vi "Keithley 6514 Zero Check Config.vi"(0 "Resource In":refnum<visa-resource-name>, 1 "Check For SCPI Errors? (T)":bool=TRUE, 7 "Zero Check (On:T)":bool=TRUE, 11 "error in (no error)":T1) -> (4 "Resource Out (dupl)":refnum<visa-resource-name>, 15 "error out":T1)   [LabVIEW 2009, in "Keithley 6514 LV 2009.lvlib"]
doc: "This VI for the Keithley 6514 Electrometer allows the operator to turn the 'Zero Check' function on or off.\n\n1 or True: Zero Check On\n0 or False: Zero Check Off"
uses:
  Keithley 6514 LV 2009.lvlib
panel:
  # "ON\nOFF"
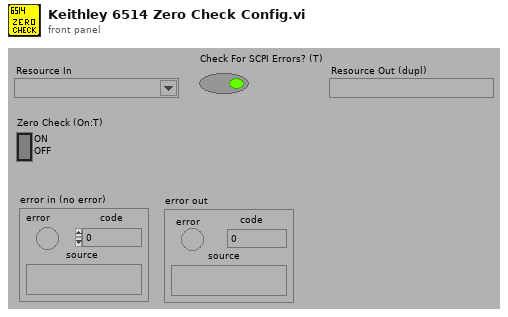
[diagram p1: front panel]
types:
  T1 = cluster{"error":bool, "code":i32, "source":string}
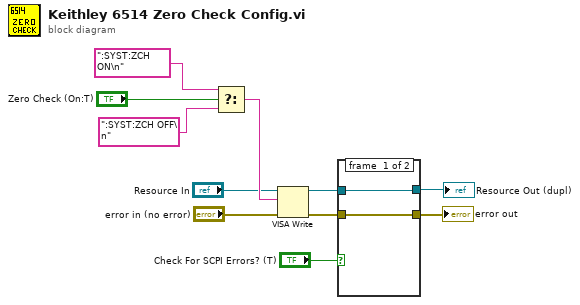
[diagram p0: block diagram]
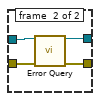
[diagram p2: hidden frame]
diagram:
  n1 = Select(t=":SYST:ZCH ON\n", s="Zero Check (On:T)", f=":SYST:ZCH OFF\n") -> (s? t:f=w8:string)
  n2 = VISA Write(VISA resource name="Resource In", write buffer=w8, error in (no error)="error in (no error)") -> (VISA resource name out=w4:refnum<visa-resource-name>, error out=w3:errorcluster)  [unwired: 1 out]
  n3 = case shown="False" "Check For SCPI Errors? (T)" {
    tunnel: w4 -> [w13 w17]
    tunnel: w3 -> [w12 w16]
    tunnel: [w13 w15] -> w2
    tunnel: [w12 w14] -> w1
    frame #0 {
    }
    frame #1 {
      n4 = call "Error Query.vi"("VISA Resource In"=w17, "error in (no error)"=w16) -> ("VISA Resource Out (dupl)"=w15:refnum<visa-resource-name>, "error out"=w14:errorcluster)  [unwired: 10 in, 2 out]
    }
  }
  "error out" <- w1
  "Resource Out (dupl)" <- w2
